vi "error_header_from_code.vi"(4 "Error/warning code":i32) -> (1 "error_header":string)   [LabVIEW 2015]
doc: "<B>Has built-in description?</B> will be True only if a description for <B>Error/warning code</B> is known by LabVIEW.\n\nSteen Schmidt\nGPower\n16/11 2012"
panel:
  # "Checks whether the error code has a BuiltIn description and therefore\nreturns appropriate error header to use when creating ones own errors\nBased on Steen Schmidt, GPower"
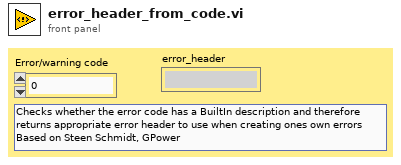
[diagram p1: front panel]
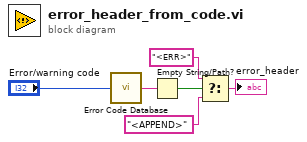
[diagram p0: block diagram]
diagram:
  n1 = call <vilib>:"Error Code Database.vi"("Error Code"="Error/warning code") -> ("Error Text"=w5:string)
  n2 = Empty String/Path?(string/path=w5) -> (empty?=w4:bool)
  n3 = Select(t="<ERR>", s=w4, f="<APPEND>") -> (s? t:f=→"error_header":string)
